vi "gjson_ArrayString.vi"(8 "error in":errorcluster, 10 "Array to Find":string, 11 "String In":string) -> (0 "error out":errorcluster, 1 "ArraySize":i32, 2 "Rest":string, 3 "Array":string)   [LabVIEW 2015, in "Json2Labv.lvlib"]
uses:
  Json2Labv.lvlib
  <vilib>/regexp/Match Regular Expression.xnode
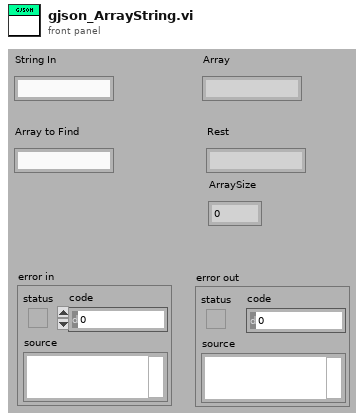
[diagram p1: front panel]
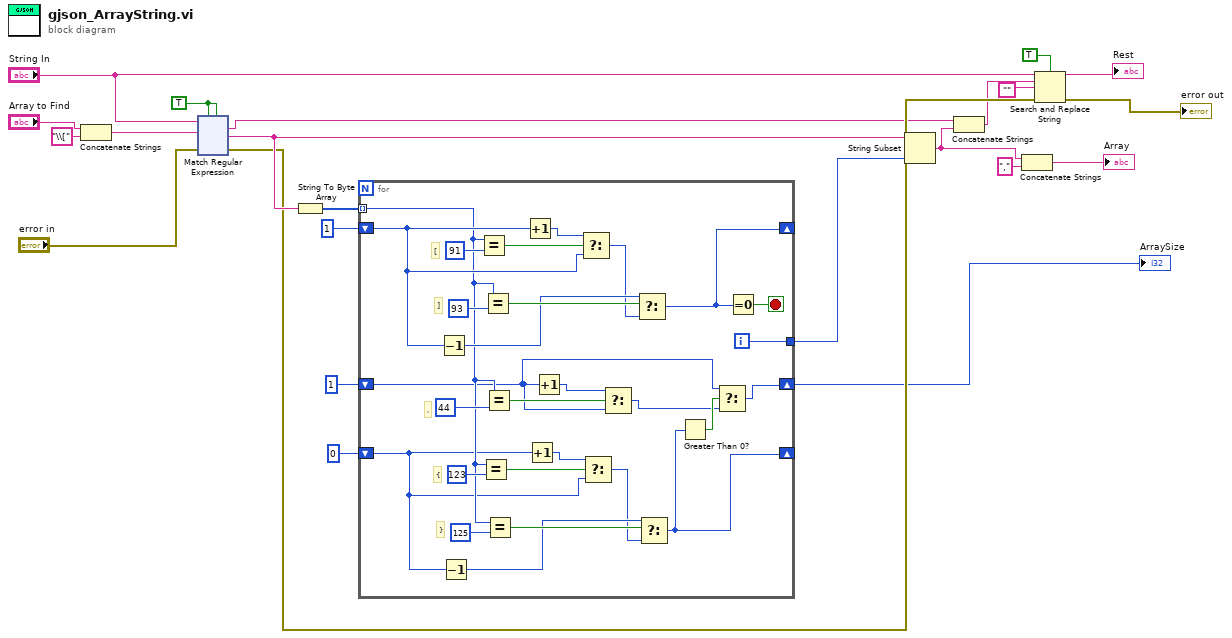
[diagram p0: block diagram]
diagram:
  w21 = TRUE ("ignore case? (F)")
  n1 = Concatenate Strings("Array to Find", "\\[" ("string")) -> (w18:string)
  n2 = xnode "Match Regular Expression"("input string"="String In", "regular expression"=w18, "error in"="error in", "ignore case? (F)"=w21, "multiline? (F)"=w21) -> ("whole match"=w4:string, "after match"=w14:string, "error out"=w10:errorcluster)  [unwired: 1 in, 2 out]
  n3 = String To Byte Array(string=w14) -> (unsigned byte array=w22:u8[])
  n4 = for {
    tunnel: w22 -> [w30] mode=indexing
    shift-right: [w43] -> _
    shift-left: 1 -> [w46]
    tunnel: [w41] -> w19
    shift-right: [w24] -> w2
    shift-left: 1 -> [w25]
    shift-right: [w28] -> _
    shift-left: 0 -> [w29]
    i -> [w41]
    stop <- w42 stop-if-true
    # "{"
    # "}"
    # ","
    # "["
    # "]"
    n5 = Decrement(x=w46) -> (x-1=w45:i32)
    n6 = Decrement(x=w29) -> (x-1=w32:i32)
    n7 = Equal?(x=w30, y=u8 91) -> (x = y?=w50:bool)
    n8 = Equal?(x=w30, y=u8 123) -> (x = y?=w36:bool)
    n9 = Equal?(x=w30, y=u8 93) -> (x = y?=w47:bool)
    n10 = Equal?(x=w30, y=u8 44) -> (x = y?=w40:bool)
    n11 = Equal?(x=w30, y=u8 125) -> (x = y?=w33:bool)
    n12 = Increment(x=w46) -> (x+1=w49:i32)
    n13 = Increment(x=w29) -> (x+1=w35:i32)
    n14 = Increment(x=w25) -> (x+1=w38:i32)
    n15 = Select(t=w49, s=w50, f=w46) -> (s? t:f=w44:i32)
    n16 = Select(t=w35, s=w36, f=w29) -> (s? t:f=w31:i32)
    n17 = Select(t=w38, s=w40, f=w25) -> (s? t:f=w26:i32)
    n18 = Select(t=w45, s=w47, f=w44) -> (s? t:f=w43:i32)
    n19 = Select(t=w32, s=w33, f=w31) -> (s? t:f=w28:i32)
    n20 = Greater Than 0?(x=w28) -> (x > 0?=w27:bool)
    n21 = Select(t=w25, s=w27, f=w26) -> (s? t:f=w24:i32)
    n22 = Equal To 0?(x=w43) -> (x = 0?=w42:bool)
  }
  "ArraySize" <- w2
  n23 = String Subset(string=w14, length (rest)=w19) -> (substring=w6:string)  [unwired: 1 in]
  n24 = Concatenate Strings(w4, w6) -> (w5:string)
  n25 = Concatenate Strings(w6, "," ("string")) -> (→"Array":string)
  n26 = Search and Replace String(case sensitive?=TRUE ("replace all? (F)"), input string="String In", search string=w5, replace string="", error in=w10) -> (result string=→"Rest":string, error out=→"error out":errorcluster)  [unwired: 3 in, 2 out]
